vi "Memory.Pointer.Error Handling.Out of Range v2.vi"(7 "source vi name":string, 8 "error in (no error)":errorcluster, 9 "value":u64 format="%d bytes", 10 "parameter":T1, 11 "Pointer in":refnum<class "Memory.Pointer.lvclass">) -> (0 "error out":errorcluster, 3 "Pointer out":refnum<class "Memory.Pointer.lvclass">)   [LabVIEW 2016, in "LabVIEW Memory Manager.lvlib" / "Memory.Pointer.lvclass"]
uses:
  Memory.Pointer.lvclass
  Typedefs/Memory.Pointer.Parameters.ctl
  Memory.Pointer.lvclass/Memory.Pointer.ctl
  Typedefs/Memory.Pointer.Error Codes.ctl
  RT Errors/VIs/Deterministic Errors.New Error Cluster (256B).vi
  Memory.Globals.vi
  RT Errors/Deterministic Error Builder.lvlib
  LabVIEW Memory Manager.lvlib
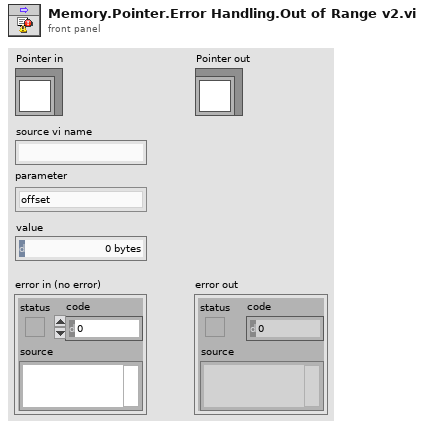
[diagram p1: front panel]
types:
  T1 = typedef "LabVIEW Memory Manager.lvlib/Memory.Pointer.lvclass/Memory.Pointer.Parameters.ctl" = enum16{"offset", "length", "size", "subset"}
  T2 = typedef "LabVIEW Memory Manager.lvlib/Memory.Pointer.lvclass/Memory.Pointer.Error Codes.ctl" = enum16{"Out of range"}
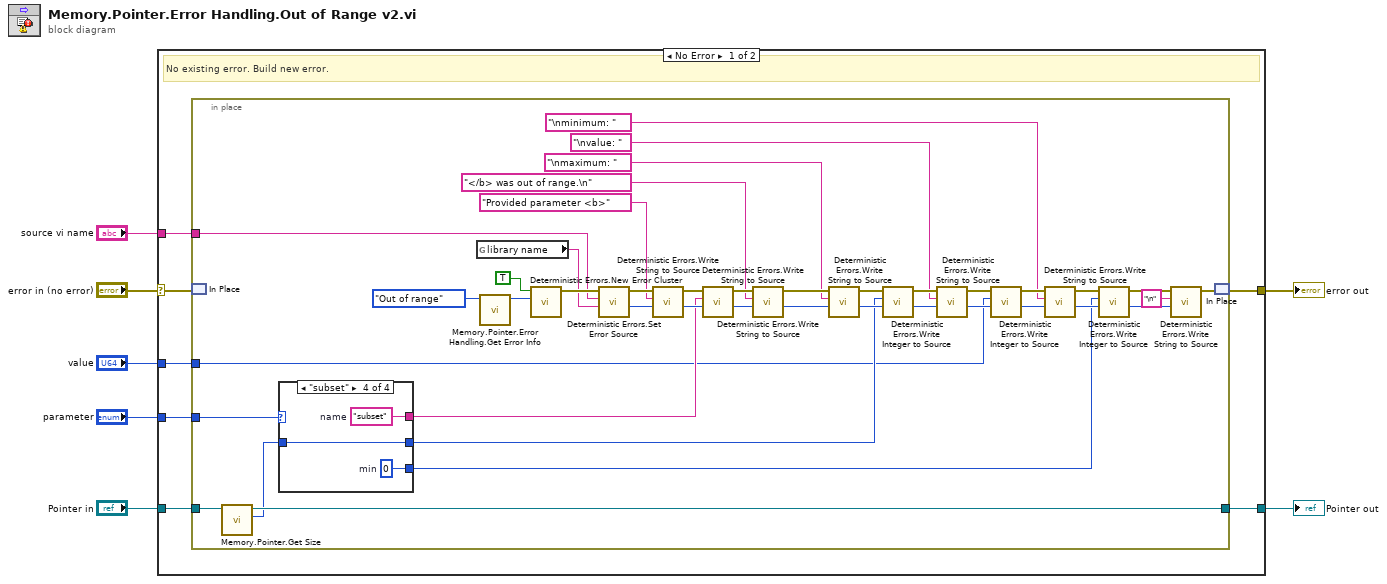
[diagram p0: block diagram]
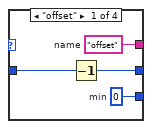
[diagram p2: hidden frame]
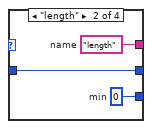
[diagram p3: hidden frame]
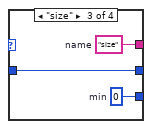
[diagram p4: hidden frame]
diagram:
  n1 = case shown="No Error" "error in (no error)" {
    selector: "error in (no error)" -> [w13 w70]
    tunnel: [w14 w70] -> w5
    tunnel: "source vi name" -> [w12 _]
    tunnel: "parameter" -> [w11 _]
    tunnel: "Pointer in" -> [w10 w69]
    tunnel: [w9 w69] -> w2
    tunnel: "value" -> [w8 _]
    frame No Error {
      # "No existing error. Build new error."
      n2 = in-place {
        in-place-border: w12 -> [w52]
        in-place-border: w11 -> [w24]
        in-place-border: w10 -> [w22]
        in-place-border: [w21] -> w9
        in-place-border: w8 -> [w16]
        n3 = in-place-match #1(w13) -> ()  [unwired: 1 out]
        n4 = call "Memory.Pointer.Get Size.vi"("Pointer in"=w22) -> ("size"=w20:i64, "Pointer out"=w21:refnum<class "Memory.Pointer.lvclass">)  [unwired: 8 in, 1 out]
        n5 = case shown="\"subset\"" w24 {
          tunnel: [w59 w62 w65 w68] -> w23
          tunnel: w20 -> [w57 w60 w63 w66]
          tunnel: [w58 w61 w64 w67] -> w15
          tunnel: [w56 w60 w63 w66] -> w17
          frame "offset" {
            w58 = 0  # min
            w59 = "offset"  # name
            n6 = Decrement(x=w57) -> (x-1=w56:i64)
          }
          frame "length" {
            w61 = 0  # min
            w62 = "length"  # name
          }
          frame "size" {
            w64 = 0  # min
            w65 = "size"  # name
          }
          frame "subset" {
            w67 = 0  # min
            w68 = "subset"  # name
          }
        }
        n7 = global read "Memory.Globals.vi" "library name"() -> (w33:string)
        n8 = call "Memory.Pointer.Error Handling.Get Error Info.vi"("error"=Memory.Pointer.Error_Codes."Out of range" ("error code")) -> ("code"=w53:i32)  [unwired: 9 in, 1 out]
        n9 = call-poly "Deterministic Errors.New Error Cluster.vi"("code (0)"=w53, "status (F)"=TRUE) -> ("error out"=w55:errorcluster)  [unwired: 9 in]
        n10 = call "Deterministic Errors.Set Error Source.vi"("library name (\"\")"=w33, "vi name"=w52, "error in"=w55) -> ("new offset"=w38:i32, "error out"=w39:errorcluster)  [unwired: 7 in]
        n11 = call "Deterministic Errors.Write String to Source.vi"("offset (0)"=w38, "string"="Provided parameter <b>", "error in"=w39) -> ("new offset"=w29:i32, "error out"=w31:errorcluster)  [unwired: 7 in]
        n12 = call "Deterministic Errors.Write String to Source.vi"("offset (0)"=w29, "string"=w23, "error in"=w31) -> ("new offset"=w28:i32, "error out"=w30:errorcluster)  [unwired: 7 in]
        n13 = call "Deterministic Errors.Write String to Source.vi"("offset (0)"=w28, "string"="</b> was out of range.\n", "error in"=w30) -> ("new offset"=w27:i32, "error out"=w26:errorcluster)  [unwired: 7 in]
        n14 = call "Deterministic Errors.Write String to Source.vi"("offset (0)"=w27, "string"="\nmaximum: ", "error in"=w26) -> ("new offset"=w48:i32, "error out"=w51:errorcluster)  [unwired: 7 in]
        n15 = call "Deterministic Errors.Write Integer to Source.vi"("offset (0)"=w48, "value"=w17, "error in"=w51) -> ("new offset"=w49:i32, "error out"=w50:errorcluster)  [unwired: 7 in]
        n16 = call "Deterministic Errors.Write String to Source.vi"("offset (0)"=w49, "string"="\nvalue: ", "error in"=w50) -> ("new offset"=w44:i32, "error out"=w45:errorcluster)  [unwired: 7 in]
        n17 = call "Deterministic Errors.Write Integer to Source.vi"("offset (0)"=w44, "value"=w16, "error in"=w45) -> ("new offset"=w42:i32, "error out"=w43:errorcluster)  [unwired: 7 in]
        n18 = call "Deterministic Errors.Write String to Source.vi"("offset (0)"=w42, "string"="\nminimum: ", "error in"=w43) -> ("new offset"=w40:i32, "error out"=w41:errorcluster)  [unwired: 7 in]
        n19 = call "Deterministic Errors.Write Integer to Source.vi"("offset (0)"=w40, "value"=w15, "error in"=w41) -> ("new offset"=w34:i32, "error out"=w37:errorcluster)  [unwired: 7 in]
        n20 = call "Deterministic Errors.Write String to Source.vi"("offset (0)"=w34, "string"="\n", "error in"=w37) -> ("error out"=w36:errorcluster)  [unwired: 7 in, 1 out]
        n21 = in-place-match #1(w36) -> (w14:errorcluster)
      }
    }
    frame Error {
      # "Incoming error. Pass through."
    }
  }
  "error out" <- w5
  "Pointer out" <- w2
